vi "EXO1_backup.vi"() -> ()   [LabVIEW 2012]
uses:
  <vilib>/FieldPoint/Polymorphic Write.llb/FP Write (Float -IO).vi
  <vilib>/FieldPoint/Polymorphic Read.llb/FP Read (Float Array -IO).vi
  <vilib>/FieldPoint/Polymorphic Read.llb/FP Read (Float -IO).vi
  <instrlib>/Dual Gauge/Dual Gauge.lvlib
panel:
  in  "V-20\n(Block)":bool
  out "Flow Speed (L/min)":dbl caption="Pressure" format="%.3e"
  out "LN2 Dewar 2":dbl(slide) scale=0.0..10.0
  out "LN2 Dewar 1":dbl(slide) scale=0.0..10.0
  out "Xenon Cell":dbl(slide) scale=0.0..10.0
  in  "Control Input 2":dbl(slide) scale=0.0..10.0
  in  "Control Input 1":dbl(slide) scale=0.0..10.0
  out "Pressure 3":dbl caption="Pressure" format="%.3e"
  out "Pressure 2":dbl caption="Pressure" format="%.3e"
  out "Pressure 1":dbl caption="Pressure" format="%.3e"
  out "Pressure 4":dbl caption="Pressure" format="%.3e"
  in  "V-10":bool
  in  "Jog":bool
  in  "Reverse / Stop":bool
  in  "Forward / Stop":bool
  in  "Speed Control Knob":dbl(knob) caption="Knob" scale=0.0..10.0 scale format="%^#_6g"
  in  "V-9":bool
  in  "V-19\n(Block)":bool
  in  "V-18\n(Block)":bool
  out "Thermocouple 1":dbl(slide) scale=0.0..100.0
  out "DT 1":dbl(slide) scale=0.0..100.0
  out "PT 1":dbl(slide) scale=0.0..100.0
  in  "V-15":bool
  in  "V-14":bool
  in  "V-7":bool
  in  "R-1":bool
  in  "V-8":bool
  in  "R-2":bool
  in  "V-2":bool
  in  "V-17\n(Proportional)":bool
  in  "V-16\n(Proportional)":bool
  in  "V-6":bool
  in  "V-4":bool
  in  "V-3":bool
  in  "V-5":bool
  in  "stop":bool
  in  "V-13":bool
  in  "V-11":bool
  in  "V-12":bool
  in  "V-1":bool
  # "EXO Front Panel"
  # "Rupture Disc"
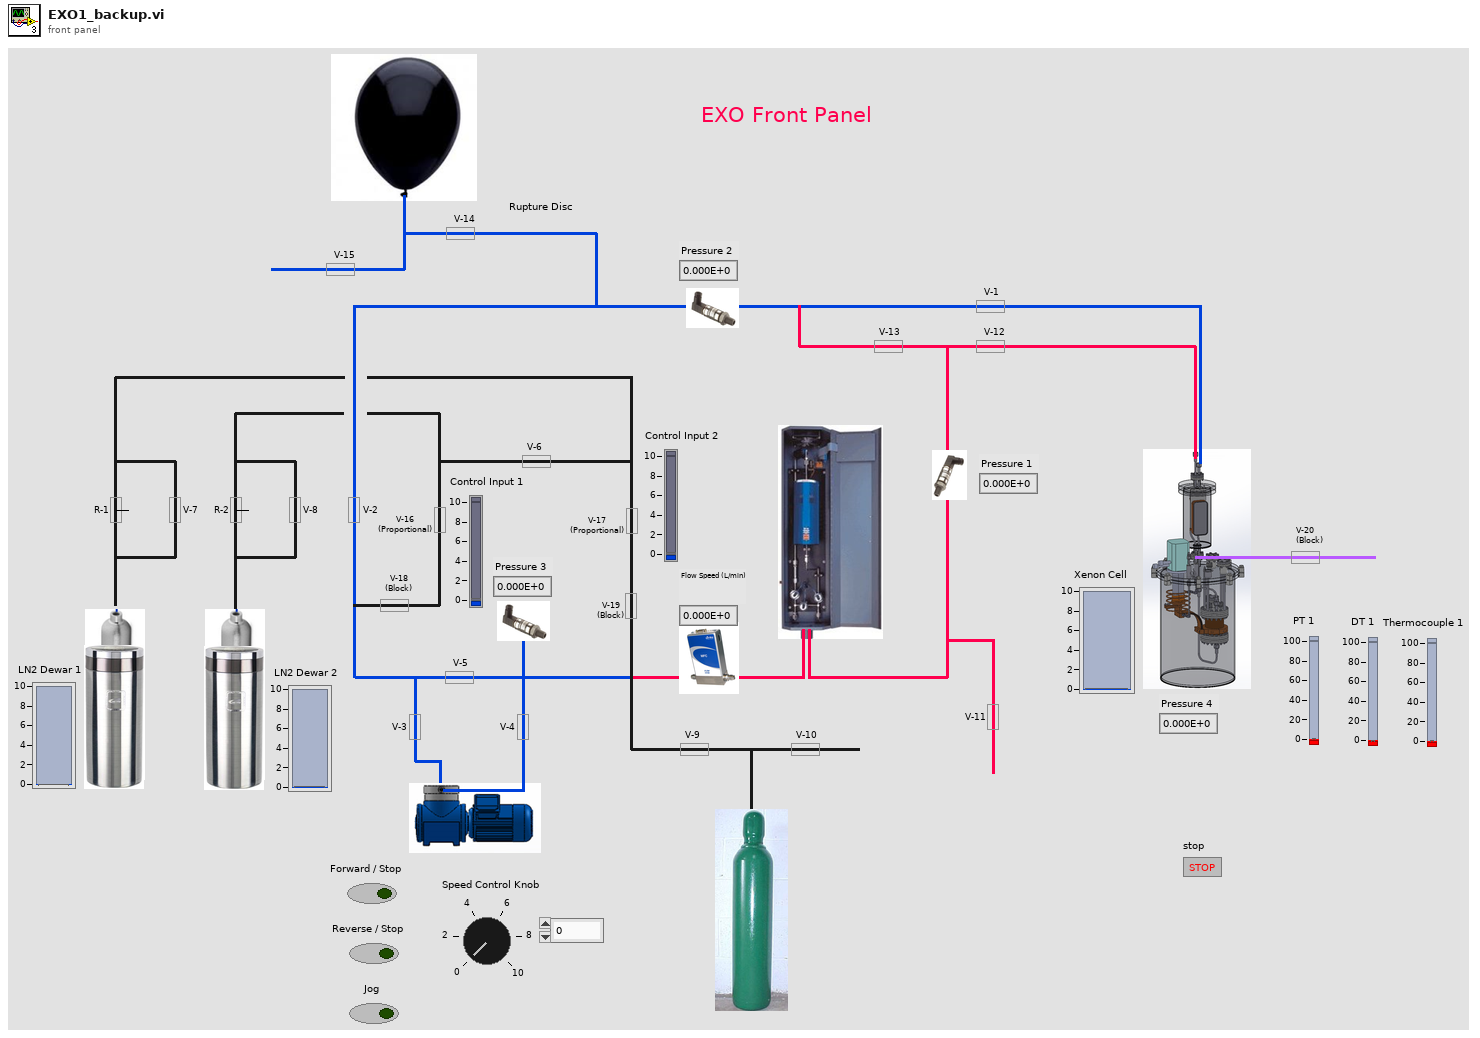
[diagram p1: front panel]
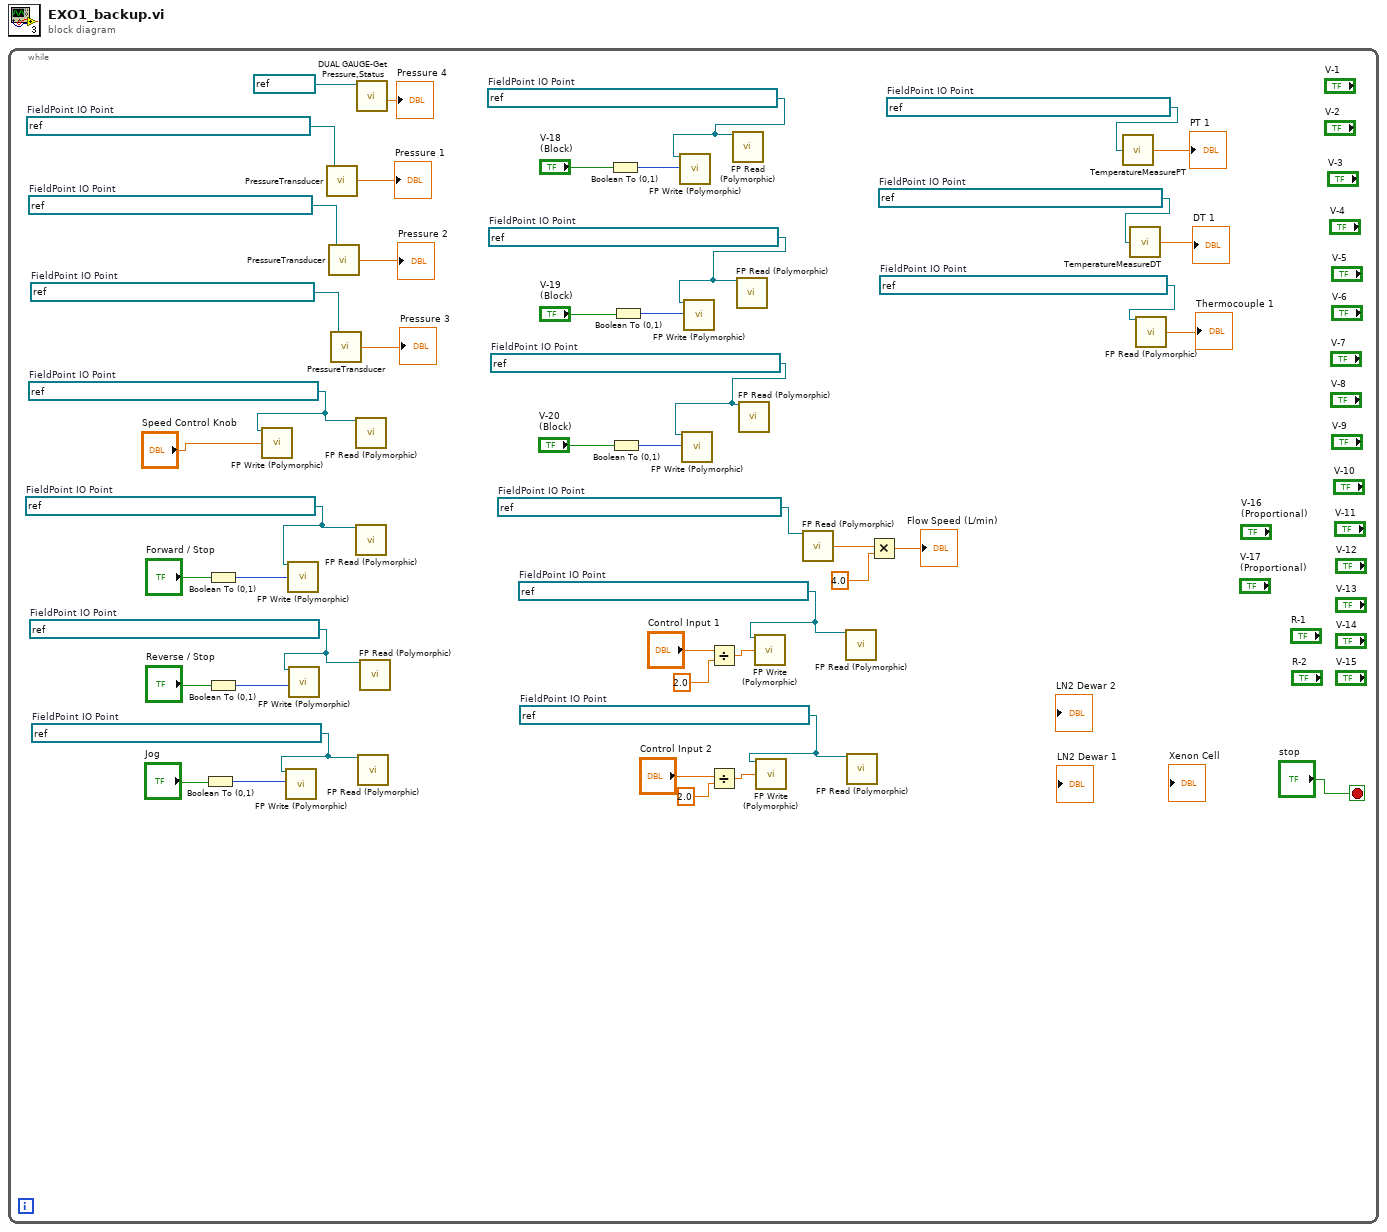
[diagram p0: block diagram]
diagram:
  n1 = while {
    stop <- "stop" stop-if-true
    w2 = refnum<k21> "FieldPoint\\Loomis434\\cFP-DO-401 @4\\Channel 5"  # FieldPoint IO Point
    w7 = refnum<k21> "FieldPoint\\Loomis434\\cFP-AI-112 @5\\Channel 2"  # FieldPoint IO Point
    w8 = refnum<k21> "FieldPoint\\Loomis434\\cFP-DO-401 @4\\Channel 4"  # FieldPoint IO Point
    w11 = refnum<k21> "FieldPoint\\Loomis434\\cFP-DO-401 @4\\Channel 3"  # FieldPoint IO Point
    w20 = refnum<k21> "FieldPoint\\Loomis434\\cFP-AO-210 @2\\Channel 2"  # FieldPoint IO Point
    w21 = refnum<k21> "FieldPoint\\Loomis434\\cFP-AO-210 @2\\Channel 1"  # FieldPoint IO Point
    w23 = refnum<k21> "FieldPoint\\Loomis434\\cFP-AI-100 @6\\Channel 1"  # FieldPoint IO Point
    w25 = refnum<k21> "FieldPoint\\Loomis434\\cFP-AI-100 @6\\Channel 1"  # FieldPoint IO Point
    w27 = refnum<k21> "FieldPoint\\Loomis434\\cFP-AI-100 @6\\Channel 0"  # FieldPoint IO Point
    w29 = refnum<k21> "FieldPoint\\Loomis434\\cFP-TC-120 @3\\Channel 0"  # FieldPoint IO Point
    w32 = refnum<k21> "FieldPoint\\Loomis434\\cFP-AI-112 @5\\Channel 1"  # FieldPoint IO Point
    w33 = refnum<k21> "FieldPoint\\Loomis434\\cFP-AI-112 @5\\Channel 0"  # FieldPoint IO Point
    w37 = refnum<k21> "FieldPoint\\Loomis434\\cFP-DO-401 @4\\Channel 2"  # FieldPoint IO Point
    w39 = refnum<k21> "FieldPoint\\Loomis434\\cFP-DO-401 @4\\Channel 1"  # FieldPoint IO Point
    w42 = refnum<k21> "FieldPoint\\Loomis434\\cFP-DO-401 @4\\Channel 0"  # FieldPoint IO Point
    w45 = refnum<k21> "FieldPoint\\Loomis434\\cFP-AO-210 @2\\Channel 0"  # FieldPoint IO Point
    n2 = Boolean To (0,1)(Boolean="Jog") -> (0, 1=w38:i16)
    n3 = Boolean To (0,1)(Boolean="Forward / Stop") -> (0, 1=w44:i16)
    n4 = Boolean To (0,1)(Boolean="Reverse / Stop") -> (0, 1=w40:i16)
    n5 = call-poly <vilib>:"FP Write (Polymorphic).vi"("FieldPoint IO Point In"=w45, "value"="Speed Control Knob") -> ()  [unwired: 11 in, 3 out]
    n6 = call-poly <vilib>:"FP Write (Polymorphic).vi"("FieldPoint IO Point In"=w37, "value"=w38) -> ()  [unwired: 11 in, 3 out]
    n7 = call-poly <vilib>:"FP Write (Polymorphic).vi"("FieldPoint IO Point In"=w42, "value"=w44) -> ()  [unwired: 11 in, 3 out]
    n8 = call-poly <vilib>:"FP Write (Polymorphic).vi"("FieldPoint IO Point In"=w39, "value"=w40) -> ()  [unwired: 11 in, 3 out]
    n9 = call "PressureTransducer.vi"("FieldPoint IO Point In"=w27) -> ("psi"=→"Pressure 1":dbl)
    n10 = call "PressureTransducer.vi"("FieldPoint IO Point In"=w25) -> ("psi"=→"Pressure 2":dbl)
    n11 = call "PressureTransducer.vi"("FieldPoint IO Point In"=w23) -> ("psi"=→"Pressure 3":dbl)
    n12 = call-poly <vilib>:"FP Read (Polymorphic).vi"("FieldPoint IO Point In"=w45) -> ()  [unwired: 11 in, 4 out]
    n13 = call-poly <vilib>:"FP Read (Polymorphic).vi"("FieldPoint IO Point In"=w42) -> ()  [unwired: 11 in, 4 out]
    n14 = call <instrlib>:"DUAL GAUGE-Get Pressure,Status.vi"("Referenz in"=refnum<visa-resource-name> "COM7") -> ("Pressure"=→"Pressure 4":dbl)  [unwired: 7 in, 3 out]
    n15 = call-poly <vilib>:"FP Read (Polymorphic).vi"("FieldPoint IO Point In"=w37) -> ()  [unwired: 11 in, 4 out]
    n16 = call-poly <vilib>:"FP Read (Polymorphic).vi"("FieldPoint IO Point In"=w39) -> ()  [unwired: 11 in, 4 out]
    n17 = Boolean To (0,1)(Boolean="V-18\n(Block)") -> (0, 1=w12:i16)
    n18 = Boolean To (0,1)(Boolean="V-20\n(Block)") -> (0, 1=w1:i16)
    n19 = Boolean To (0,1)(Boolean="V-19\n(Block)") -> (0, 1=w9:i16)
    n20 = call-poly <vilib>:"FP Write (Polymorphic).vi"("FieldPoint IO Point In"=w11, "value"=w12) -> ()  [unwired: 11 in, 3 out]
    n21 = call-poly <vilib>:"FP Write (Polymorphic).vi"("FieldPoint IO Point In"=w2, "value"=w1) -> ()  [unwired: 11 in, 3 out]
    n22 = call-poly <vilib>:"FP Write (Polymorphic).vi"("FieldPoint IO Point In"=w8, "value"=w9) -> ()  [unwired: 11 in, 3 out]
    n23 = Divide(x="Control Input 1", y=2.0) -> (x/y=w18:dbl)
    n24 = Divide(x="Control Input 2", y=2.0) -> (x/y=w16:dbl)
    n25 = call-poly <vilib>:"FP Read (Polymorphic).vi"("FieldPoint IO Point In"=w11) -> ()  [unwired: 11 in, 4 out]
    n26 = call-poly <vilib>:"FP Read (Polymorphic).vi"("FieldPoint IO Point In"=w8) -> ()  [unwired: 11 in, 4 out]
    n27 = call-poly <vilib>:"FP Read (Polymorphic).vi"("FieldPoint IO Point In"=w2) -> ()  [unwired: 11 in, 4 out]
    n28 = call-poly <vilib>:"FP Write (Polymorphic).vi"("FieldPoint IO Point In"=w21, "value"=w18) -> ()  [unwired: 11 in, 3 out]
    n29 = call-poly <vilib>:"FP Write (Polymorphic).vi"("FieldPoint IO Point In"=w20, "value"=w16) -> ()  [unwired: 11 in, 3 out]
    n30 = call-poly <vilib>:"FP Read (Polymorphic).vi"("FieldPoint IO Point In"=w7) -> ("value"=w5:dbl)  [unwired: 11 in, 3 out]
    n31 = call-poly <vilib>:"FP Read (Polymorphic).vi"("FieldPoint IO Point In"=w21) -> ()  [unwired: 11 in, 4 out]
    n32 = call-poly <vilib>:"FP Read (Polymorphic).vi"("FieldPoint IO Point In"=w20) -> ()  [unwired: 11 in, 4 out]
    n33 = Multiply(x=w5, y=4.0) -> (x*y=→"Flow Speed (L/min)":dbl)
    n34 = call "TemperatureMeasurePT.vi"("FieldPoint IO Point In"=w33) -> ("Ch1 [K]"=→"PT 1":dbl)
    n35 = call "TemperatureMeasureDT.vi"("FieldPoint IO Point In"=w32) -> ("Ch2 [K]"=→"DT 1":dbl)
    n36 = call-poly <vilib>:"FP Read (Polymorphic).vi"("FieldPoint IO Point In"=w29) -> ("value"=→"Thermocouple 1":dbl)  [unwired: 11 in, 3 out]
  }
